vi "Close Child.vi"(8 "error in (no error)":errorcluster, 11 "Websocket Client in":refnum<class "Websocket Client.lvclass">) -> (0 "error out":errorcluster, 3 "Websocket Client out":refnum<class "Websocket Client.lvclass">)   [LabVIEW 2020, in "Stream-Websocket.lvlib" / "Websocket Client.lvclass"]
uses:
  Websocket Client.lvclass
  Websocket Client.lvclass/Websocket Client.ctl
  <vilib>/IlluminatedG/lv-stream/Connection/Connection.lvclass
  C:/Program Files (x86)/National Instruments/LabVIEW 2020/vi.lib/IlluminatedG/lv-stream/Connection/Connection.lvclass
  C:/Program Files (x86)/National Instruments/LabVIEW 2020/vi.lib/IlluminatedG/lv-stream/Endpoint/Endpoint.lvclass
  C:/dev/IlluminatedG/lv-stream-websocket/Stream-Websocket/Websocket Client/Websocket Client.lvclass
  Client Command.ctl
  Stream-Websocket.lvlib
  <vilib>/IlluminatedG/lv-stream/Connection/State.ctl
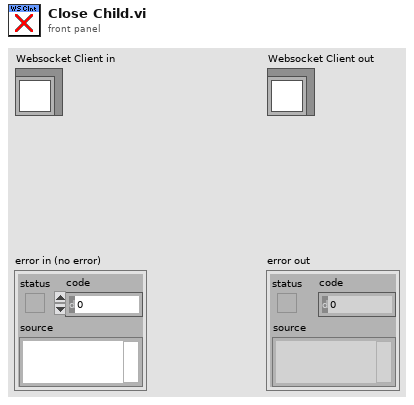
[diagram p1: front panel]
types:
  T1 = typedef "Stream.lvlib/Connection.lvclass/State.ctl" = enum16{"Closed", "Idle", "Connecting", "Connected", "Shutdown"}
  T2 = typedef "Stream-Websocket.lvlib/Client Command.ctl" = enum16{"Connect", "Close", "Shutdown", "Reconnect"}
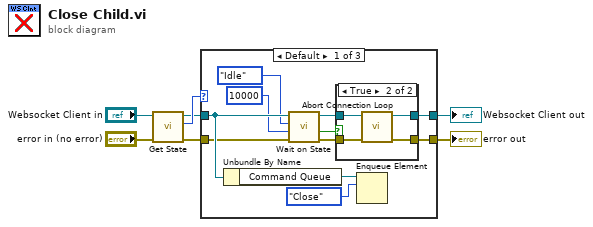
[diagram p0: block diagram]
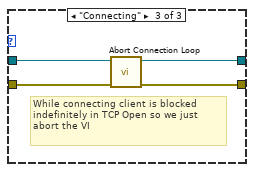
[diagram p4: hidden frame]
diagram:
  n1 = call <vilib>:"Get State.vi"("error in (no error)"="error in (no error)", "Connection in"="Websocket Client in") -> ("error out"=w3:errorcluster, "State"=w5:T1, "Connection out"=w4:refnum<class "Websocket Client.lvclass">)  [unwired: 7 in]
  n2 = case shown="Default" w5 {
    tunnel: w4 -> [w16 w26 w30]
    tunnel: w3 -> [w15 w25 w29]
    tunnel: [w9 w26 w28] -> w2
    tunnel: [w8 w25 w27] -> w1
    frame Default {
      n3 = Unbundle By Name(w16) -> ("Command Queue"=w18:refnum<queue>)
      n4 = call <vilib>:"Wait on State.vi"("error in (no error)"=w15, "Timeout ms (-1)"=10000, "State"=State."Idle", "Connection in"=w16) -> ("error out"=w11:errorcluster, "Timed Out?"=w12:bool, "Connection out"=w10:refnum<class "Websocket Client.lvclass">)  [unwired: 5 in]
      n5 = case shown="True" w12 {
        tunnel: w11 -> [w19 w23]
        tunnel: w10 -> [w20 w24]
        tunnel: [w20 w22] -> w9
        tunnel: [w19 w21] -> w8
        frame False {
        }
        frame True {
          n6 = call "Abort Connection Loop.vi"("error in (no error)"=w23, "Websocket Client in"=w24) -> ("error out"=w21:errorcluster, "Websocket Client out"=w22:refnum<class "Websocket Client.lvclass">)  [unwired: 8 in]
        }
      }
      n7 = Enqueue Element(queue=w18, element=Client_Command."Close") -> ()  [unwired: 2 in, 3 out]
    }
    frame "Closed", "Idle" {
    }
    frame "Connecting" {
      # "While connecting client is blocked indefinitely in TCP Open so we just abort the VI"
      n8 = call "Abort Connection Loop.vi"("error in (no error)"=w29, "Websocket Client in"=w30) -> ("error out"=w27:errorcluster, "Websocket Client out"=w28:refnum<class "Websocket Client.lvclass">)  [unwired: 8 in]
    }
  }
  "error out" <- w1
  "Websocket Client out" <- w2
